vi "Write.vi"(8 "error in (no error)":errorcluster, 10 "Message":refnum<class "Message Interface.lvclass">, 11 "Websocket Client Handler in":refnum<class "Websocket Client Handler.lvclass">) -> (0 "error out":errorcluster, 3 "Websocket Client Handler out":refnum<class "Websocket Client Handler.lvclass">)   [LabVIEW 2016, in "Stream Mediator.lvlib" / "Websocket Client Handler.lvclass"]
doc: "--\nCopyright © 2017 Composed SystemsI All rights reserved.\n\nAuthor: Jon McBee <jon.mcbee@composed.io>\n\nThis library is provided \"AS IS\" ,WITHOUT WARRANTIES OR\nCONDITIONS OF ANY KIND, either express or implied.\n\nComposed Systems -- composed.io\n\nStream 0.0.1.1\nJon McBee - Composed Systems\nCopyright (c) 2017, Composed Systems"
uses:
  <userlib>/Composed Systems/Stream/Mediator/Classes/Websocket Client Handler Actor/Websocket Client Handler/Websocket Client Handler.lvclass
  C:/Program Files (x86)/National Instruments/LabVIEW 2016/user.lib/Composed Systems/Stream/Mediator/Classes/Mediated Asynchronous Actor/Mediated Asynchronous Actor.lvclass
  <userlib>/Composed Systems/Stream/Mediator/Classes/Message Interface/Message Interface.lvclass
  <userlib>/Composed Systems/Stream/Mediator/Classes/Mediated Asynchronous Actor/Mediated Asynchronous Actor.lvclass
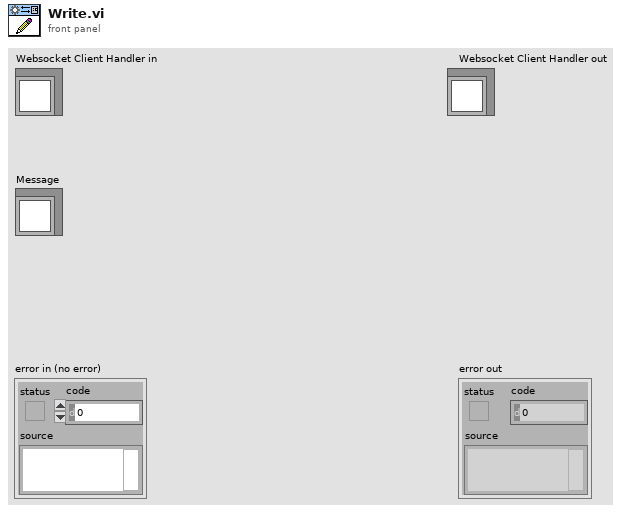
[diagram p1: front panel]
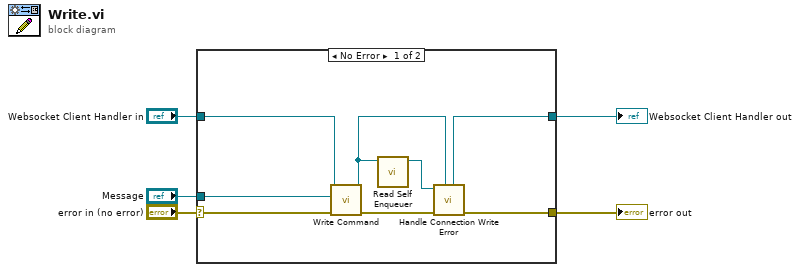
[diagram p0: block diagram]
diagram:
  n1 = case shown="No Error" "error in (no error)" {
    selector: "error in (no error)" -> [w13 w15]
    tunnel: [w9 w15] -> w4
    tunnel: [w8 w14] -> w2
    tunnel: "Websocket Client Handler in" -> [w12 w14]
    tunnel: "Message" -> [w11 _]
    frame No Error {
      n2 = call <userlib>:"Write Command.vi"("error in (no error)"=w13, "Message"=w11, "Websocket Client Handler in"=w12) -> ("error out"=w10:errorcluster, "Websocket Client Handler out"=w7:refnum<class "Websocket Client Handler.lvclass">)  [unwired: 7 in]
      n3 = call <userlib>:"Read Self Enqueuer.vi"("Mediated Asynchronous Actor in"=w7) -> ("Self Enqueuer"=w6:refnum<class "Message Transport Queue.lvclass">)  [unwired: 10 in]
      n4 = call-dynamic "Handle Connection Write Error.vi"("Websocket Client Handler in"=w7, "error in (no error)"=w10, "Self Enqueuer"=w6) -> ("error out"=w9:errorcluster, "Websocket Client Handler out"=w8:refnum<class "Websocket Client Handler.lvclass">)  [unwired: 7 in]
    }
    frame Error {
    }
  }
  "error out" <- w4
  "Websocket Client Handler out" <- w2
